vi "Ultrasonic SRF06 calib.vi"(1 "Sensor offset (m)":dbl=0.27, 2 "Ambient temperature (deg C)":dbl=20.0, 3 "Sensor Voltage (V)":dbl=4.072) -> (0 "Distance (m)":dbl=0.9999999999999998)   [LabVIEW 2011]
panel:
  in  "T0 (K)":dbl=293.15
  in  "1/G (A/m)-1":dbl=318.75
  in  "I0 (A)":dbl=0.004
  in  "R (ohm)":dbl=510.0
  # "by Paul Nathan 02/04/2012. Specifically for Devantech SRF06 ultrasonic rangers installed in ENFLO lab towing tank."
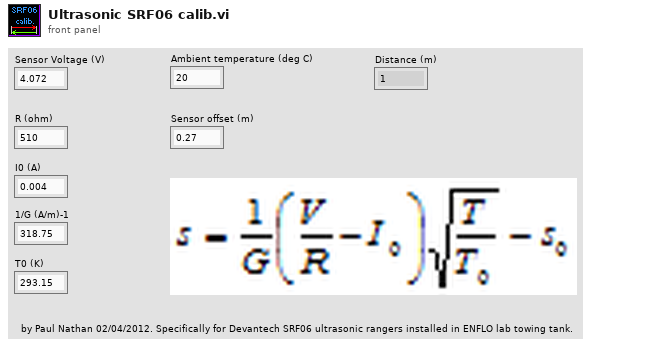
[diagram p1: front panel]
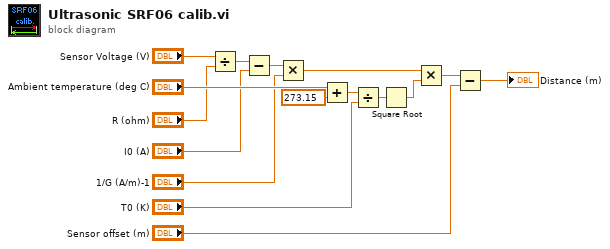
[diagram p0: block diagram]
diagram:
  n1 = Divide(x="Sensor Voltage (V)", y="R (ohm)") -> (x/y=w9:dbl)
  n2 = Subtract(x=w9, y="I0 (A)") -> (x-y=w7:dbl)
  n3 = Multiply(x=w7, y="1/G (A/m)-1") -> (x*y=w4:dbl)
  n4 = Add(x="Ambient temperature (deg C)", y=273.15) -> (x+y=w14:dbl)
  n5 = Divide(x=w14, y="T0 (K)") -> (x/y=w12:dbl)
  n6 = Square Root(x=w12) -> (sqrt(x)=w5:dbl)
  n7 = Multiply(x=w4, y=w5) -> (x*y=w3:dbl)
  n8 = Subtract(x=w3, y="Sensor offset (m)") -> (x-y=→"Distance (m)":dbl)
